vi "getDesiredForbarVal.vi"(1 "inputVal":dbl) -> (0 "outputVal":dbl)   [LabVIEW 2018]
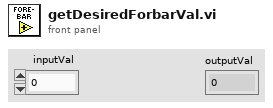
[diagram p1: front panel]
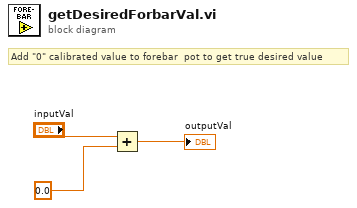
[diagram p0: block diagram]
diagram:
  # "Add \"0\" calibrated value to forebar  pot to get true desired value"
  n1 = Add(x="inputVal", y=0.0) -> (x+y=→"outputVal":dbl)
